vi "NMR12.vi"() -> ()   [LabVIEW 2013]
uses:
  <vilib>/Analysis/NI_AALBase.lvlib
panel:
  in  "AutoBaseline":bool
  out "RF OK":bool
  out "Peak area (V-MHz)":sgl=0.025455328 format="%.3f"
  in  "Gauss Fit":bool
  out "NMR Graph + Fit":cluster{cluster{dbl, "Numeric":dbl}[]}[](graph)=[{[{224.21, "Numeric"=-0.0179017968749825}, {224.215, "Numeric"=-0.02089154296876572}, {224.22, "Numeric"=-0.01778755859379766}, {224.225, "Numeric"=-0.015315917968828363}, {224.23000000000002, "Numeric"=-0.019458066406164543}, {224.235, "Numeric"=-0.0070206445311966625}, {224.24, "Numeric"=-0.00780101562497737}, {224.245, "Numeric"=-0.017831894531256776}, {224.25, "Numeric"=-0.027677246093784746}, {224.255, "Numeric"=-0.017744785156311504}, {224.26000000000002, "Numeric"=-0.01833236328116894}, {224.26500000000001, "Numeric"=-0.021212441406197047}, {224.27, "Numeric"=-0.021599863281223985}, {224.275, "Numeric"=-0.01699218749999959}, {224.28, "Numeric"=-0.023698007812523847}, {224.285, "Numeric"=-0.01593607421879678}, {224.29000000000002, "Numeric"=-0.010454433593675205}, {224.29500000000002, "Numeric"=-0.020998203124949655}, {224.3, "Numeric"=-0.016671386718722758}, {224.305, "Numeric"=-0.019092636718744505}, {224.31, "Numeric"=-0.01550560546876495}, {224.315, "Numeric"=-0.005653945312533992}, {224.32000000000002, "Numeric"=-0.024510800781183506}, {224.32500000000002, "Numeric"=-0.02745947265620416}, {224.33, "Numeric"=-0.015317832031223416}, {224.335, "Numeric"=-0.014611757812491383}, {224.34, "Numeric"=-0.014000917968757992}, {224.345, "Numeric"=-0.008687949218773278}, {224.35, "Numeric"=0.001461425781212805}, {224.35500000000002, "Numeric"=-0.012495664062460637}, {224.36, "Numeric"=-0.008237441406226093}, {224.365, "Numeric"=-0.015964101562490174}, {224.37, "Numeric"=-0.01281187500000297}, {224.375, "Numeric"=-0.008888183593764448}, {224.38, "Numeric"=-0.014373691406274577}, {224.38500000000002, "Numeric"=-0.012300624999969062}, {224.39000000000001, "Numeric"=-0.005085976562480693}, {224.395, "Numeric"=0.003632558593759022}, {224.4, "Numeric"=-0.005932617187499954}, {224.405, "Numeric"=0.011469960937492404}, {224.41, "Numeric"=0.012810507812486091}, {224.41500000000002, "Numeric"=0.018950839843770523}, {224.42000000000002, "Numeric"=0.009200039062512714}, {224.425, "Numeric"=0.015955566406256238}, {224.43, "Numeric"=0.02720570312500109}, {224.435, "Numeric"=0.04379273437499727}, {224.44, "Numeric"=0.07451792968749478}, {224.44500000000002, "Numeric"=0.12430072265625815}, {224.45000000000002, "Numeric"=0.19472802734375416}, {224.455, "Numeric"=0.3284512109375015}, {224.46, "Numeric"=0.6074893164062501}, {224.465, "Numeric"=1.01649810546875}, {224.47, "Numeric"=1.1187466210937516}, {224.475, "Numeric"=0.7778090820312542}, {224.48000000000002, "Numeric"=0.4645473046874936}, {224.485, "Numeric"=0.28583384765624475}, {224.49, "Numeric"=0.18140259765624728}, {224.495, "Numeric"=0.12707142578125108}, {224.5, "Numeric"=0.09654638671875625}, {224.505, "Numeric"=0.05382894531251271}, {224.51000000000002, "Numeric"=0.05245914062498111}, {224.51500000000001, "Numeric"=0.02415083984373609}, {224.52, "Numeric"=0.021760488281242413}, {224.525, "Numeric"=0.0032592773437500402}, {224.53, "Numeric"=-0.007536874999990985}, {224.535, "Numeric"=-0.02137015624998069}, {224.54000000000002, "Numeric"=-0.018318691406283394}, {224.54500000000002, "Numeric"=-0.016802890625024575}, {224.55, "Numeric"=-0.024806152343764445}, {224.555, "Numeric"=-0.025494980468752967}, {224.56, "Numeric"=-0.022629140624990177}, {224.565, "Numeric"=-0.02504652343747607}, {224.57000000000002, "Numeric"=-0.03723931640629985}, {224.57500000000002, "Numeric"=-0.03712500000003721}, {224.58, "Numeric"=-0.04324605468752327}, {224.585, "Numeric"=-0.027282167968757987}, {224.59, "Numeric"=-0.02908929687499137}, {224.595, "Numeric"=-0.0326396093749734}, {224.6, "Numeric"=-0.041290039062454154}, {224.60500000000002, "Numeric"=-0.04273589843755182}, {224.61, "Numeric"=-0.030934707031284037}, {224.615, "Numeric"=-0.02300072265626496}, {224.62, "Numeric"=-0.035022812499994505}, {224.625, "Numeric"=-0.030501953124972725}, {224.63, "Numeric"=-0.036610996093699666}, {224.63500000000002, "Numeric"=-0.030303066406318413}, {224.64000000000001, "Numeric"=-0.03091410156254676}, {224.645, "Numeric"=-0.03473316406252386}, {224.65, "Numeric"=-0.04520263671874958}, {224.655, "Numeric"=-0.04255933593747402}, {224.66, "Numeric"=-0.032674843749947}, {224.66500000000002, "Numeric"=-0.030173183593836916}, {224.67000000000002, "Numeric"=-0.037398105468811504}, {224.675, "Numeric"=-0.03541650390628481}, {224.68, "Numeric"=-0.03121080078125671}, {224.685, "Numeric"=-0.040991933593727325}, {224.69, "Numeric"=-0.03894203124994666}, {224.69500000000002, "Numeric"=-0.03155523437510743}, {224.70000000000002, "Numeric"=-0.03489599609382832}, {224.705, "Numeric"=-0.030446250000047637}, {224.71, "Numeric"=-0.02797162109376572}]}]
  in  "Amp of Q curve":dbl=14.599999999999989 format="%_3f"
  in  "Subtract Q curve":bool=TRUE
  in  "Adjust Tune":bool
  out "IF Offset":dbl(graph)=3.047351611328092
  out "Pedestal Difference":dbl(graph)=-0.017865110677106836
  out "# Good Spectra":i32=987
  in  "Quality cuts":bool=TRUE
  out "Pedestal OK":bool=TRUE
  out "Sweep #":i32=1
  out "1st Sweep":bool
  out "ADC volts OK":bool=TRUE
  out "Peak Height Distribution":cluster{"Y":dbl[], "Y":dbl[]}[](graph)=[{"Y"=[0.9620044397786442, 0.9625205367838526, 0.9630366337890609, 0.9635527307942693, 0.9640688277994777, 0.9645849248046859, 0.9651010218098943, 0.9656171188151026, 0.966133215820311, 0.9666493128255192, 0.9671654098307276, 0.967681506835936, 0.9681976038411443, 0.9687137008463527, 0.9692297978515609, 0.9697458948567693, 0.9702619918619776, 0.970778088867186, 0.9712941858723944, 0.9718102828776026, 0.972326379882811, 0.9728424768880193, 0.9733585738932277, 0.9738746708984359, 0.9743907679036443, 0.9749068649088527, 0.975422961914061, 0.9759390589192694, 0.9764551559244776, 0.976971252929686, 0.9774873499348943, 0.9780034469401027, 0.978519543945311, 0.9790356409505193, 0.9795517379557277, 0.980067834960936, 0.9805839319661444, 0.9811000289713526, 0.981616125976561, 0.9821322229817694, 0.9826483199869777, 0.983164416992186, 0.9836805139973943, 0.9841966110026027, 0.984712708007811, 0.9852288050130193, 0.9857449020182276, 0.986260999023436, 0.9867770960286444, 0.9872931930338527, 0.987809290039061, 0.9883253870442693, 0.9888414840494777, 0.989357581054686, 0.9898736780598943, 0.9903897750651027, 0.990905872070311, 0.9914219690755194, 0.9919380660807277, 0.992454163085936, 0.9929702600911443, 0.9934863570963527, 0.9940024541015611, 0.9945185511067693, 0.9950346481119777, 0.995550745117186, 0.9960668421223944, 0.9965829391276027, 0.997099036132811, 0.9976151331380194, 0.9981312301432277, 0.9986473271484361, 0.9991634241536443, 0.9996795211588527, 1.000195618164061, 1.0007117151692695, 1.0012278121744778, 1.001743909179686, 1.0022600061848943, 1.0027761031901028, 1.003292200195311, 1.0038082972005193, 1.0043243942057278, 1.004840491210936, 1.0053565882161444, 1.0058726852213526, 1.0063887822265611, 1.0069048792317694, 1.0074209762369777, 1.0079370732421862, 1.0084531702473944, 1.0089692672526027, 1.009485364257811, 1.0100014612630195, 1.0105175582682278, 1.011033655273436, 1.0115497522786443, 1.0120658492838528, 1.012581946289061, 1.0130980432942693], "Y"=[1.0, 1.0, 0.0, 2.0, 0.0, 1.0, 2.0, 0.0, 3.0, 6.0, 2.0, 3.0, 3.0, 5.0, 4.0, 4.0, 3.0, 4.0, 4.0, 10.0, 10.0, 7.0, 15.0, 8.0, 11.0, 7.0, 8.0, 10.0, 13.0, 12.0, 17.0, 14.0, 18.0, 12.0, 8.0, 19.0, 16.0, 21.0, 17.0, 23.0, 13.0, 20.0, 25.0, 20.0, 17.0, 25.0, 18.0, 19.0, 23.0, 21.0, 14.0, 19.0, 20.0, 14.0, 21.0, 22.0, 15.0, 14.0, 24.0, 21.0, 13.0, 12.0, 20.0, 15.0, 11.0, 14.0, 13.0, 14.0, 9.0, 8.0, 13.0, 13.0, 6.0, 9.0, 10.0, 3.0, 9.0, 9.0, 4.0, 9.0, 8.0, 8.0, 10.0, 7.0, 4.0, 3.0, 4.0, 1.0, 6.0, 1.0, 2.0, 0.0, 1.0, 1.0, 4.0, 2.0, 1.0, 0.0, 0.0, 1.0]}]
  in  "# of Sweeps":i32=1000
  out "Std Dev (V)":dbl=0.009783462944979376 format="%_2g"
  out "Peak mean (V)":dbl=0.9871274161736019 format="%_4g"
  out "Peak Height":dbl(graph)=1.1187466210937516
  in  "Raw Data":bool=TRUE
  in  "Tank RF ON":bool=TRUE
  in  "IF Atten (dB)":i8 min=0 max=35 step=5
  in  "IFoffset (V)":dbl=3.047351611328092 min=0.0 max=3000.0 step=0.001 format="%.3f"
  in  "Tune  (V)":dbl=2.0659999999999745 min=0.0 max=5.0 step=0.001 format="%.3f"
  in  "Hi / Lo Gain":bool
  out "Voltage Array":sgl[](array[numeric])=[0.9129394, 0.8734497, 0.8407837, 0.8082153, 0.7697632, 0.7486206, 0.71499026, 0.67283934, 0.631604, 0.61087644, 0.58035886, 0.5482788, 0.5194214, 0.49628907, 0.46257323, 0.44405517, 0.42398682, 0.38862306, 0.36885986, 0.3430786, 0.32403564, 0.3119873, 0.27196044, 0.24857178, 0.24100342, 0.22272949, 0.20509033, 0.1928833, 0.18624267, 0.15622559, 0.1451538, 0.12282715, 0.11210938, 0.10289307, 0.08499756, 0.07539062, 0.07165527, 0.07015381, 0.051098634, 0.05974121, 0.05305176, 0.05189209, 0.03557129, 0.036486816, 0.042626955, 0.054833986, 0.08190918, 0.12877198, 0.19700928, 0.32927245, 0.60758054, 1.0165894, 1.1195679, 0.78009033, 0.46901855, 0.2932251, 0.19244385, 0.14249268, 0.117077634, 0.080200195, 0.08540039, 0.06439209, 0.07003174, 0.060290527, 0.058984376, 0.055371094, 0.06937256, 0.08256836, 0.0869751, 0.09942627, 0.11616211, 0.12834473, 0.13148193, 0.14765625, 0.1583252, 0.19180909, 0.20825195, 0.22368164, 0.23474121, 0.25373536, 0.28670654, 0.31654054, 0.32714844, 0.35502928, 0.37301025, 0.40413818, 0.42907715, 0.4515381, 0.4680786, 0.4984619, 0.5368164, 0.56851804, 0.5912231, 0.62386477, 0.6594604, 0.6817993, 0.71669924, 0.757666, 0.78863525, 0.828125, 0.8663696] format="%.4f"
  in  "Invert Polarity":bool=TRUE
  out "Pedestal Diff (V)":sgl=-0.01786511 format="%.3f"
  out "Peak amp (V)":sgl=1.1187466 format="%.3f"
  in  "Save Data to File":bool
  in  "RF Level (dBm)":dbl min=-10.0 max=1.0 step=0.1 format="%.2f"
  out "SMT error out":errorcluster
  out "Sample RMS (V)":dbl=0.011689130171150124 format="%.4f"
  in  "# Sample/step":i32=100 min=1 max=1000 step=100
  in  "ADC Rate (Hz)":i32=10000 min=1 max=20000 step=1000
  in  "ADC Range":i32(ring)=1 items=["+- 10 V"=1, "+- 2.5 V"=3]
  in  "Step Width (MHz)":dbl=0.005 min=0.0 max=1000.0 step=0.0005 format="%.4f"
  in  "Freq Span (MHz)":dbl=0.5 min=0.0 max=3000.0 step=0.1 format="%.3f"
  in  "Center Freq (MHz)":dbl=224.46 min=0.005 max=6000.0 step=0.1 format="%.3f"
  in  "Sweep Mode":u16(ring)=3 items=["Off", "Single", "Auto", "Step"]
  in  "GPIB Addr (28)":refnum<visa-resource-name>="GPIB0::28::INSTR"
  # "Settings"
  # "E1039 Prototype NMR Control Panel"
  # "D\nA\nC"
  # "R\nF\n\nG\ne\nn\ne\nr\na\nt\no\nr"
  # "A\nD\nC"
  # "D\na\nt\na"
  # "I\n/\nO"
  # "Results"
  # "A\nv\ne\nr\na\ng\ne"
  # "S\nw\ne\ne\np"
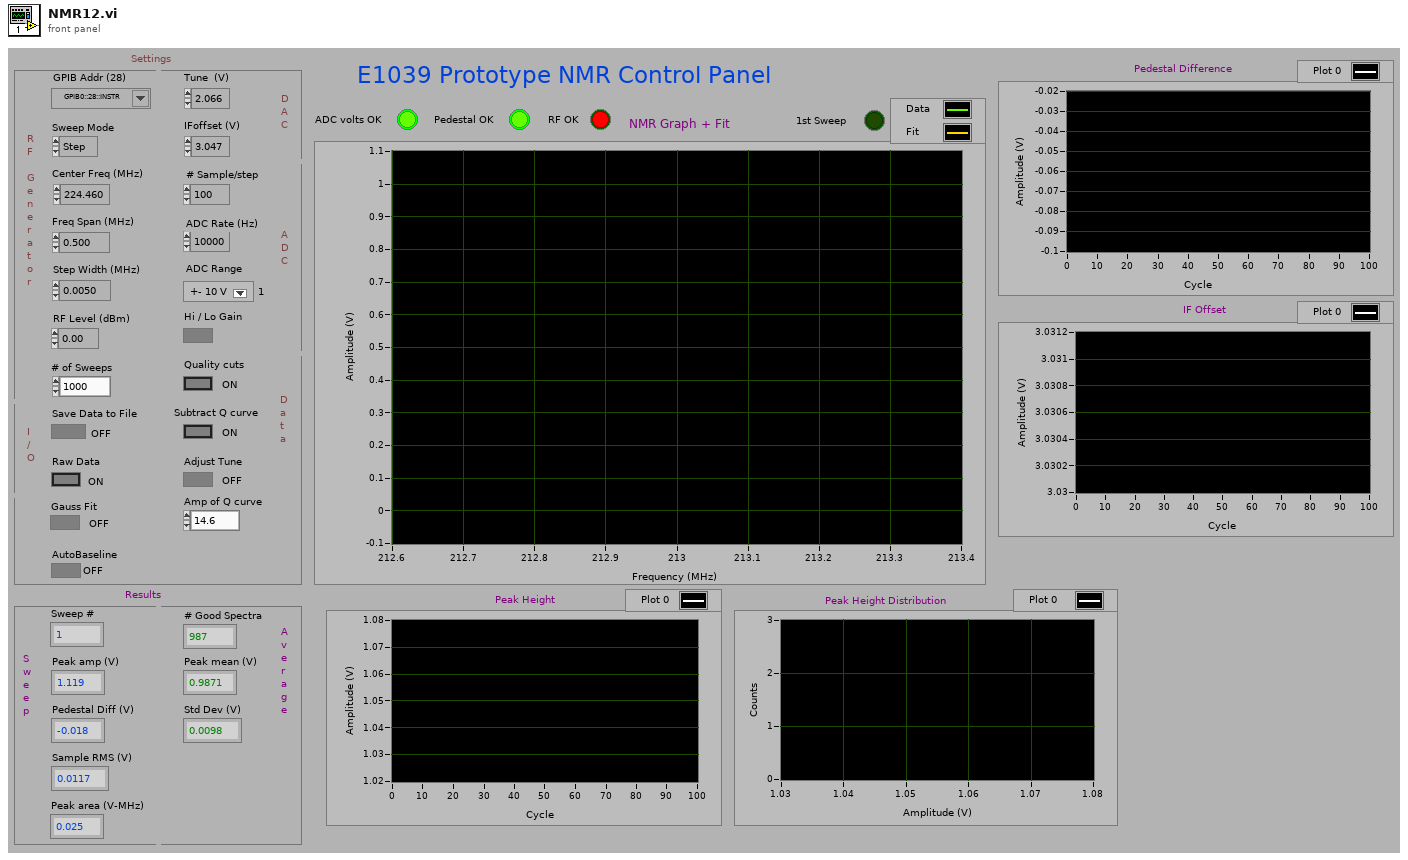
[diagram p1: front panel]
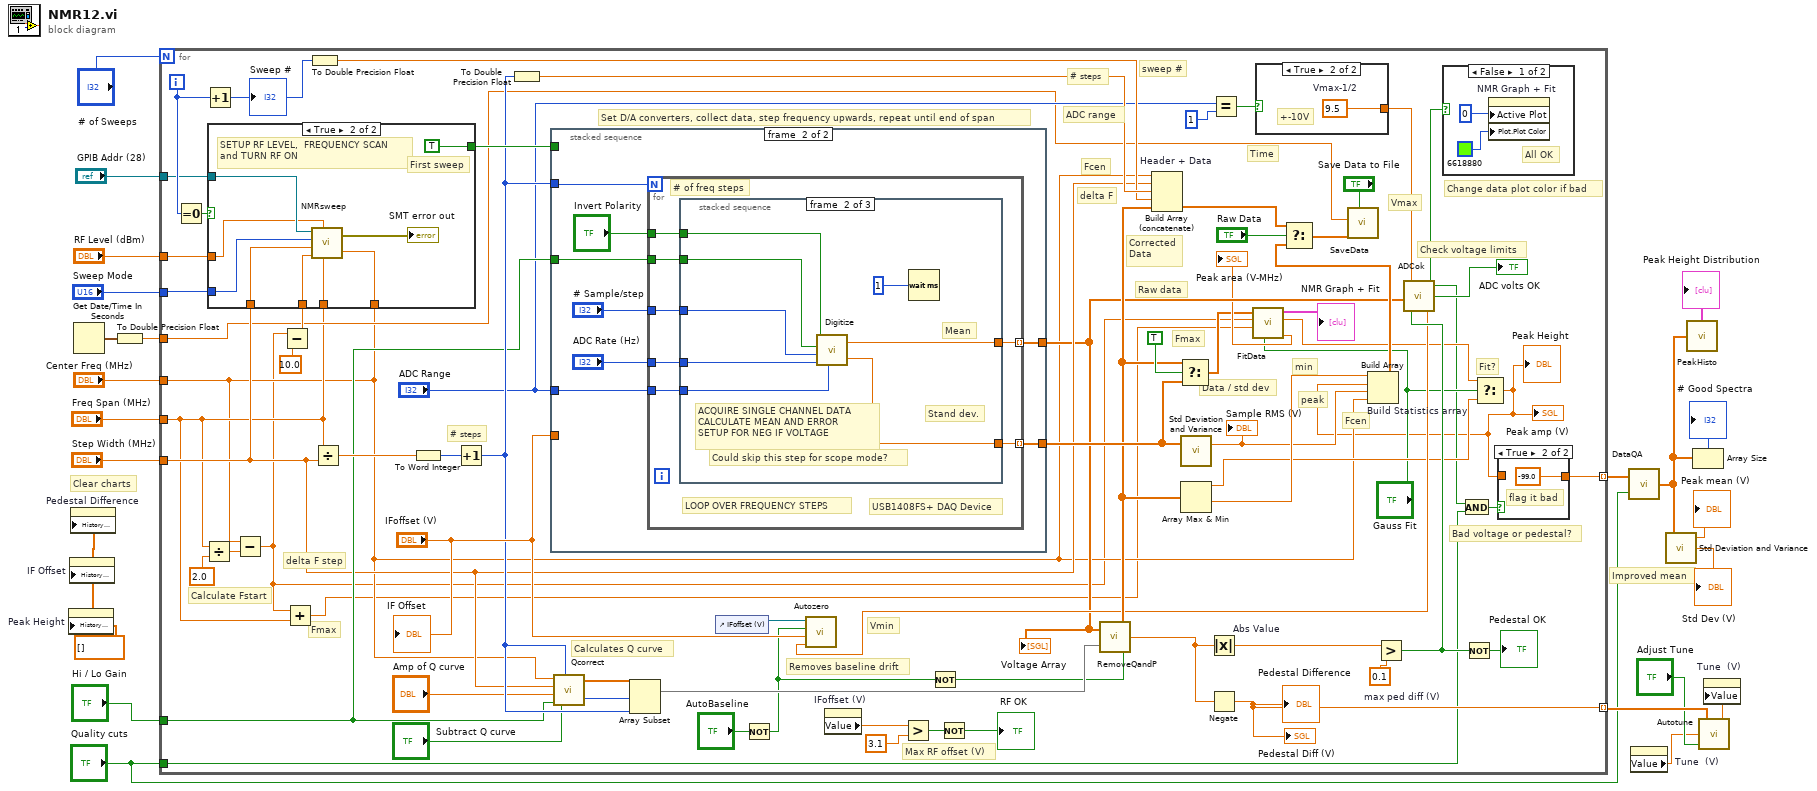
[diagram p0: block diagram]
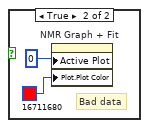
[diagram p2: hidden frame]
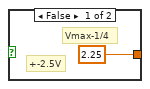
[diagram p3: hidden frame]
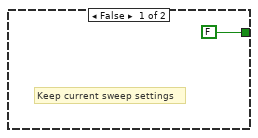
[diagram p5: hidden frame]
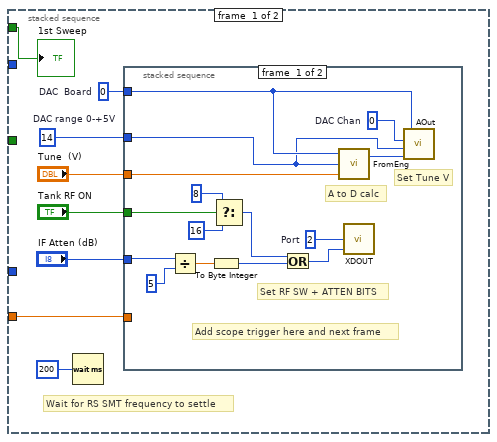
[diagram p6: hidden frame]
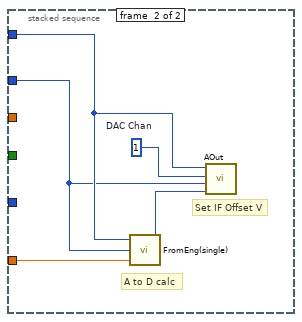
[diagram p7: hidden frame]
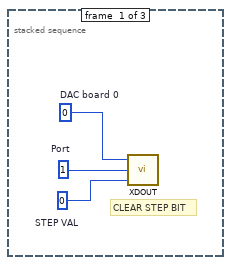
[diagram p8: hidden frame]
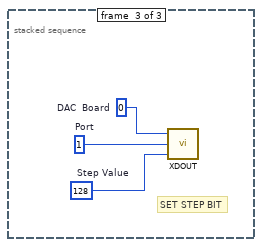
[diagram p9: hidden frame]
diagram:
  w6 = dbl[] []
  # "Clear charts"
  # "Improved mean"
  n1 = property on="Peak Height" class="WFChart (strict)"("History Data"=w6) -> ()  [unwired: 2 in, 2 out]
  n2 = property on="IF Offset" class="WFChart (strict)"("History Data"=w6) -> ()  [unwired: 2 in, 2 out]
  n3 = property on="Pedestal Difference" class="WFChart (strict)"("History Data"=w6) -> ()  [unwired: 2 in, 2 out]
  n4 = Get Date/Time In Seconds() -> (seconds since 1Jan1904=w2:timestamp)
  n5 = To Double Precision Float(number=w2) -> (double precision float=w1:dbl)
  n6 = for {
    N: "# of Sweeps" -> [_]
    tunnel: [w76] -> w18 mode=indexing
    tunnel: "Quality cuts" -> [w48]
    tunnel: [w57] -> w15 mode=indexing
    tunnel: "Center Freq (MHz)" -> [w35]
    tunnel: "Freq Span (MHz)" -> [w41]
    tunnel: "Step Width (MHz)" -> [w47]
    tunnel: "Sweep Mode" -> [w61]
    tunnel: "Hi / Lo Gain" -> [w60]
    tunnel: "GPIB Addr (28)" -> [w59]
    tunnel: "RF Level (dBm)" -> [w58]
    tunnel: w1 -> [w42]
    i -> [w74]
    w77 = 0.1  # max ped diff (V)
    # "Vmax"
    # "Change data plot color if bad"
    # "Max RF offset (V)"
    # "Fmax"
    # "Fit?"
    # "Fmax"
    # "Time"
    # "Vmin"
    # "min"
    # "peak"
    # "Raw data"
    # "Corrected\nData"
    # "Fcen"
    # "delta F"
    # "# steps"
    # "ADC range"
    # "sweep #"
    # "Fcen"
    # "Set D/A converters, collect data, step frequency upwards, repeat until end of span"
    # "Calculates Q curve"
    # "Removes baseline drift"
    # "Bad voltage or pedestal?"
    # "Check voltage limits"
    # "Data / std dev"
    # "# steps"
    # "Calculate Fstart"
    # "delta F step"
    n7 = Equal To 0?(x=w74) -> (x = 0?=w79:bool)
    n8 = Divide(x=w41, y=sgl 2.0) -> (x/y=w91:dbl)
    n9 = Increment(x=w74) -> (x+1=w64:i32)
    "Sweep #" <- w64
    n10 = Subtract(x=w35, y=w91) -> (x-y=w30:dbl)
    n11 = Subtract(x=w30, y=10.0) -> (x-y=w89:dbl)
    n12 = case shown="True" w79 {
      tunnel: w89 -> [_ w111]
      tunnel: w47 -> [_ w109]
      tunnel: w35 -> [_ w108]
      tunnel: w41 -> [_ w110]
      tunnel: [FALSE TRUE] -> w78
      tunnel: w61 -> [_ w105]
      tunnel: w59 -> [_ w104]
      tunnel: w58 -> [_ w103]
      frame False {
        # "Keep current sweep settings"
      }
      frame True {
        # "First sweep"
        # "SETUP RF LEVEL,  FREQUENCY SCAN\nand TURN RF ON"
        n13 = call "NMRsweep.vi"("Center Freq (MHz)"=w108, "Freq Span (MHz)"=w110, "RF Level (dBm)"=w103, "Foffset (MHz)"=w111, "Step Width (MHz)"=w109, "Sweep Mode"=w105, "GPIB Addr (28)"=w104) -> ("error out"=→"SMT error out":errorcluster)
      }
    }
    n14 = Add(x=w30, y=w41) -> (x+y=w29:dbl)
    n15 = To Double Precision Float(number=w64) -> (double precision float=w65:dbl)
    n16 = Divide(x=w41, y=w47) -> (x/y=w93:dbl)
    n17 = To Word Integer(number=w93) -> (16bit integer=w90:i16)
    n18 = Increment(x=w90) -> (x+1=w68:i16)
    n19 = To Double Precision Float(number=w68) -> (double precision float=w67:dbl)
    n20 = stacked-sequence {
      tunnel: [_ w147] -> w82
      tunnel: [_ w146] -> w45
      tunnel: w68 -> [_ w145]
      tunnel: "IFoffset (V)" -> [w113 _]
      tunnel: w60 -> [_ w144]
      tunnel: w78 -> [w112 _]
      tunnel: "ADC Range" -> [_ w143]
      frame #0 {
        w117 = 14  # DAC range 0-+5V
        w118 = 0  # DAC  Board
        # "Wait for RS SMT frequency to settle"
        n21 = Wait (ms)(milliseconds to wait=200) -> ()  [unwired: 1 out]
        n22 = stacked-sequence {
          tunnel: w118 -> [w125 w137]
          tunnel: w117 -> [w124 w136]
          tunnel: "Tune  (V)" -> [w123 _]
          tunnel: "Tank RF ON" -> [w121 _]
          tunnel: "IF Atten (dB)" -> [w120 _]
          tunnel: w113 -> [_ w135]
          frame #0 {
            w127 = 2  # Port
            w134 = 0  # DAC Chan
            # "Add scope trigger here and next frame"
            # "A to D calc"
            # "Set RF SW + ATTEN BITS"
            # "Set Tune V"
            n23 = Divide(x=w120, y=5) -> (x/y=w132:dbl)
            n24 = To Byte Integer(number=w132) -> (8bit integer=w129:i8)
            n25 = Select(t=8, s=w121, f=16) -> (s? t:f=w128:i32)
            n26 = Or(x=w128, y=w129) -> (x .or. y?=w126:i32)
            n27 = call-poly "FromEng.VI"("Eng Units"=w123, "Range"=w124, "BoardNum (0)"=w125) -> ("DA Data"=w122:u16)  [unwired: 1 out]
            n28 = call "XDOUT.VI"(2:w126, "PortNum"=w127) -> ()  [unwired: 3 in]
            n29 = call "AOut.VI"("DataValue"=w122, "Range"=w124, "Channel"=w134, "BoardNum"=w125) -> ()  [unwired: 1 out]
          }
          frame #1 {
            w139 = 1  # DAC Chan
            # "A to D calc"
            # "Set IF Offset V"
            n30 = call "FromEng(single).VI"("Eng Units"=w135, "Range"=w136, "BoardNum (0)"=w137) -> ("DA Data"=w138:u16)  [unwired: 1 out]
            n31 = call "AOut.VI"("DataValue"=w138, "Range"=w136, "Channel"=w139, "BoardNum"=w137) -> ()  [unwired: 1 out]
          }
        }
        "1st Sweep" <- w112
      }
      frame #1 {
        n32 = for {
          N: w145 -> [_]
          tunnel: [w154] -> w146 mode=indexing
          tunnel: [w153] -> w147 mode=indexing
          tunnel: w144 -> [w152]
          tunnel: w143 -> [w151]
          tunnel: "ADC Rate (Hz)" -> [w150]
          tunnel: "# Sample/step" -> [w149]
          tunnel: "Invert Polarity" -> [w148]
          # "# of freq steps"
          # "USB1408FS+ DAQ Device"
          # "LOOP OVER FREQUENCY STEPS"
          n33 = stacked-sequence {
            tunnel: [_ w164 _] -> w154
            tunnel: [_ w163 _] -> w153
            tunnel: w152 -> [_ w162 _]
            tunnel: w151 -> [_ w161 _]
            tunnel: w150 -> [_ w160 _]
            tunnel: w149 -> [_ w159 _]
            tunnel: w148 -> [_ w158 _]
            frame #0 {
              w155 = 0  # DAC board 0
              w156 = 0  # STEP VAL
              w157 = 1  # Port
              # "CLEAR STEP BIT"
              n34 = call "XDOUT.VI"(2:w156, "PortNum"=w157, "BoardNum"=w155) -> ()  [unwired: 2 in]
            }
            frame #1 {
              # "Could skip this step for scope mode?"
              # "Stand dev."
              # "Mean"
              # "ACQUIRE SINGLE CHANNEL DATA\nCALCULATE MEAN AND ERROR\nSETUP FOR NEG IF VOLTAGE"
              n35 = call "Digitize.vi"("Invert Polarity"=w158, "IF or Log"=w162, "# Sample/step"=w159, "ADC Rate (Hz)"=w160, "ADC Range"=w161) -> ("mean"=w164:dbl, "standard deviation"=w163:dbl)
              n36 = Wait (ms)(milliseconds to wait=1) -> ()  [unwired: 1 out]
            }
            frame #2 {
              w166 = 128  # Step Value
              w168 = 0  # DAC  Board
              w167 = 1  # Port
              # "SET STEP BIT"
              n37 = call "XDOUT.VI"(2:w166, "PortNum"=w167, "BoardNum"=w168) -> ()  [unwired: 2 in]
            }
          }
        }
      }
    }
    "Voltage Array" <- w45
    n38 = call "Qcorrect.vi"("Subtract Q curve"="Subtract Q curve", "Nstep"=w68, "IF or Log"=w60, "Amp of Q curve"="Amp of Q curve", "Step Width (MHz)"=w47, "Center Freq (MHz)"=w35) -> ("Start"=w84:i32, "Array"=w85:dbl[])
    n39 = Array Subset "Array Subset"(array=w85, index=w84, length=w68) -> (w83:dbl[])
    n40 = control-ref of="IFoffset (V)"() -> (w51:refnum<vi>)
    n41 = Not(x="AutoBaseline") -> (.not. x?=w24:bool)
    n42 = property on="IFoffset (V)" class="DigNum (strict)"() -> ("Value"=w39:dbl)  [unwired: 2 in, 2 out]
    n43 = Greater?(x=w39, y=3.1) -> (0:w37:bool)
    n44 = Not(x=w24) -> (.not. x?=w23:bool)
    n45 = Not(x=w37) -> (.not. x?=→"RF OK":bool)
    n46 = call "RemoveQandP.vi"("Raw data"=w45, "Qcurve"=w83, "Subtract Ped?"=w23) -> ("Corrected data"=w66:dbl[], "Ped L-R"=w70:dbl)
    n47 = Build Array (concatenate) "Header + Data"(w35, w47, w67, w65, w66) -> (w69:dbl[])
    n48 = Select(t=w66, s=TRUE, f=w82) -> (s? t:f=w31:dbl[])
    n49 = call <vilib>:"Std Deviation and Variance.vi"("X"=w82) -> ("mean"=w46:dbl)  [unwired: 1 in, 2 out]
    "Sample RMS (V)" <- w46
    n50 = Array Max & Min(array=w66) -> (max value=w40:dbl, min value=w81:dbl)  [unwired: 2 out]
    n51 = Absolute Value "Abs Value"(x=w70) -> (abs(x)=w72:dbl)
    n52 = Negate(x=w70) -> (-x=w57:dbl)
    "Pedestal Diff (V)" <- w57
    "Pedestal Difference" <- w57
    n53 = Equal?(x="ADC Range", y=1) -> (x = y?=w55:bool)
    n54 = call "FitData.vi"("Fit?"="Gauss Fit", "Fmax"=w29, "Fmin"=w30, "Yarray"=w31) -> ("Peak Area (V-MHz)"=→"Peak area (V-MHz)":dbl, "Amplitude (V)"=w33:dbl, "NMR Graph + Fit"=→"NMR Graph + Fit":cluster{cluster{dbl, "Numeric":dbl}[]}[])  [unwired: 2 out]
    n55 = case shown="True" w55 {
      tunnel: [2.25 w99] -> w52
      frame False {
        # "Vmax-1/4"
        # "+-2.5V"
      }
      frame True {
        w99 = 9.5  # Vmax-1/2
        # "+-10V"
      }
    }
    n56 = Greater?(x=w72, y=w77) -> (0:w56:bool)
    n57 = call "ADCok.vi"("PedOK"=w56, "Array"=w45, "Vmax-1/2"=w52) -> ("Vmin"=w50:dbl, "ADC voltages OK"=→"ADC volts OK":bool, "Allok"=w27:bool)
    n58 = call "Autozero.vi"("Vmin (V)"=w50, "IFoffset (V)"="IFoffset (V)", "IF or Log"=w24, "reference"=w51) -> ()
    n59 = case shown="False" w27 {
      frame False {
        # "All OK"
        n60 = property on="NMR Graph + Fit" class="XYGraph (strict)"("Active Plot"=0, "Plot.Plot Color"=u32 6618880) -> ()  [unwired: 2 in, 2 out]
      }
      frame True {
        # "Bad data"
        n61 = property on="NMR Graph + Fit" class="XYGraph (strict)"("Active Plot"=0, "Plot.Plot Color"=u32 16711680) -> ()  [unwired: 2 in, 2 out]
      }
    }
    n62 = And(x=w27, y=w48) -> (x .and. y?=w73:bool)
    n63 = Not(x=w56) -> (.not. x?=→"Pedestal OK":bool)
    n64 = Select(t=w33, s="Gauss Fit", f=w40) -> (s? t:f=w26:dbl)
    "Peak amp (V)" <- w26
    "Peak Height" <- w26
    n65 = Build Array "Build Statistics array"(w81, w26, w46, w35) -> (w88:dbl[])
    n66 = Select(t=w69, s="Raw Data", f=w88) -> (s? t:f=w43:dbl[])
    n67 = call "SaveData.vi"("Array"=w43, "Save Data to File"="Save Data to File", "Ext time (sec)"=w42) -> ()  [unwired: 1 out]
    n68 = case shown="True" w73 {
      tunnel: [w100 -99.0] -> w76
      tunnel: w26 -> [w100 _]
      frame False {
        # "Data OK"
      }
      frame True {
        # "flag it bad"
      }
    }
    "IF Offset" <- "IFoffset (V)"
  }
  n69 = call "DataQA.vi"("Quality cuts"="Quality cuts", "Data In"=w18) -> ("Data Out"=w17:dbl[])
  n70 = property on="Tune  (V)" class="DigNum (strict)"() -> ("Value"=w5:dbl)  [unwired: 2 in, 2 out]
  n71 = call <vilib>:"Std Deviation and Variance.vi"("X"=w17) -> ("mean"=→"Peak mean (V)":dbl, "standard deviation"=→"Std Dev (V)":dbl)  [unwired: 1 in, 1 out]
  n72 = call "PeakHisto.vi"("Data Out"=w17) -> ("XY Graph"=→"Peak Height Distribution":cluster{"Y":dbl[], "Y":dbl[]}[])
  n73 = Array Size(array=w17) -> (size(s)=→"# Good Spectra":i32)
  n74 = call "Autotune.vi"("Adjust Tune"="Adjust Tune", "Tune Vin"=w5, "Pedestal Diff"=w15) -> ("Tune Vout"=w4:dbl)
  n75 = property on="Tune  (V)" class="DigNum (strict)"("Value"=w4) -> ()  [unwired: 2 in, 2 out]
